vi "Read_Camera_Variant.vi"(8 "error in (no error)":errorcluster, 9 "Variant":variant, 10 "input cluster in":T1 {"Image Type" items=["Grayscale (U8)", "Grayscale (U16)"]; "ROI Parameters"."Size(um)" min=0 max=255 step=0.1 format="%.2f"; "ROI Parameters"."Count" min=0 max=255 step=0.1 format="%.2f"}) -> (0 "error out":errorcluster, 1 "Pixel Size":dbl, 2 "Gain":dbl, 3 "Exposure":dbl, 5 "input cluster out":T1 {"Image Type" items=["Grayscale (U8)", "Grayscale (U16)"]; "ROI Parameters"."Size(um)" min=0 max=255 step=0.1 format="%.2f"; "ROI Parameters"."Count" min=0 max=255 step=0.1 format="%.2f"})   [LabVIEW 2023, in "Camera_Controller.lvlib"]
uses:
  typedefs/ImageProcessingParameters.ctl
  <vilib>/vision/Image Controls.llb/IMAQ Image.ctl
  typedefs/Image Type.ctl
  Camera_Controller.lvlib
  <userlib>/_OpenG.lib/lvdata/lvdata.llb/openg_variant.lvlib
  typedefs/typedefs.lvlib
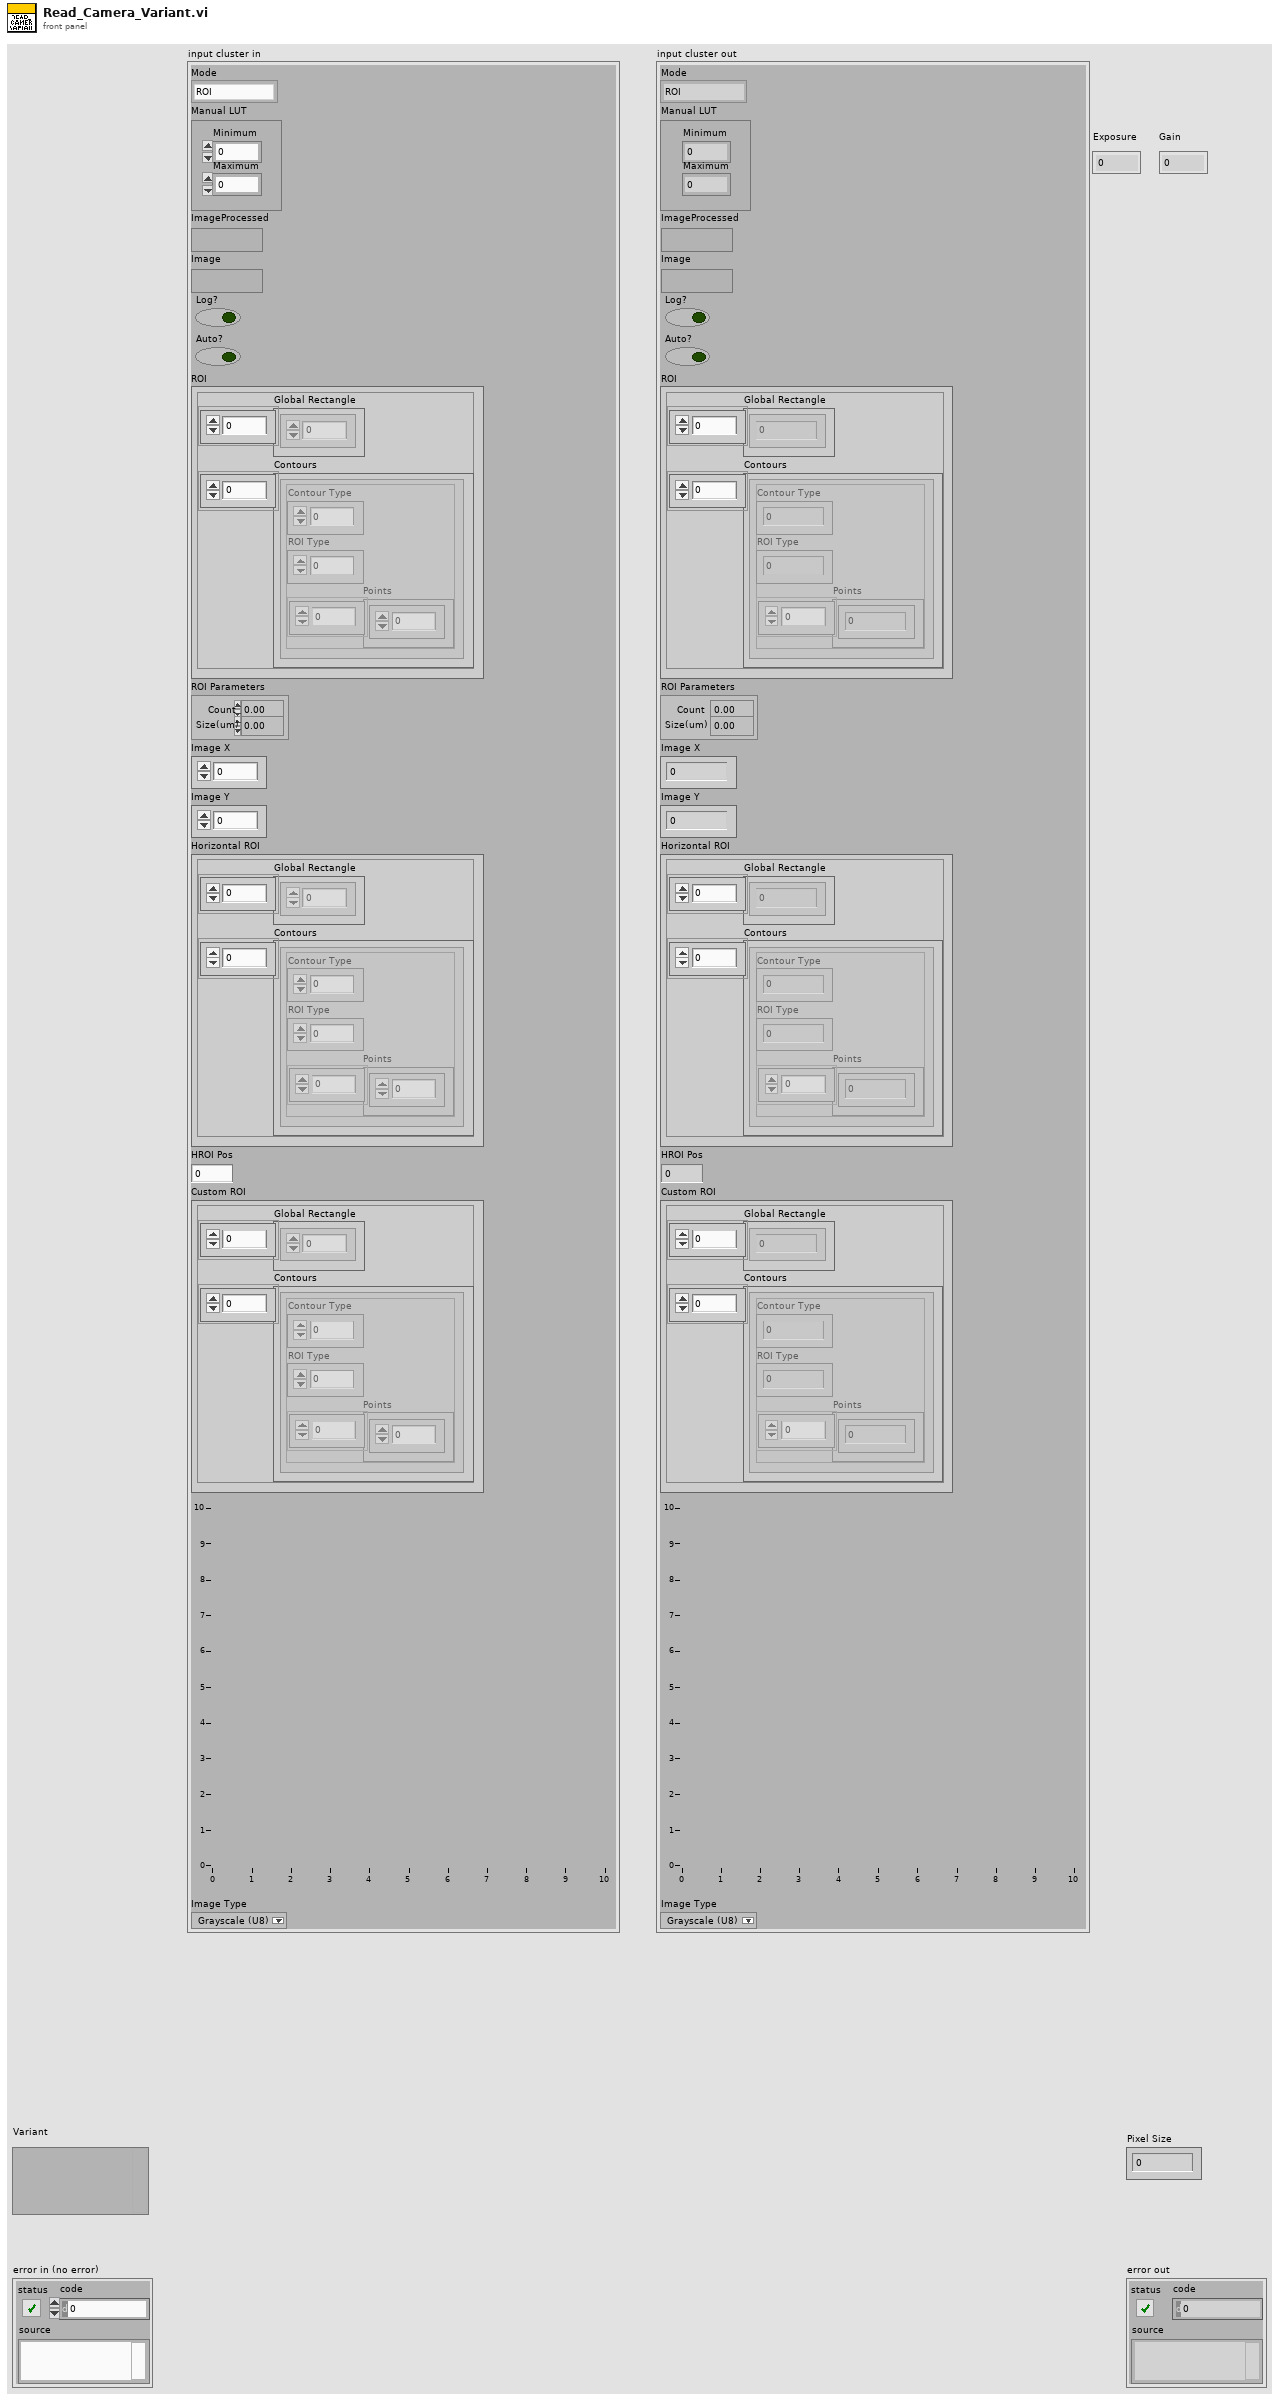
[diagram p1: front panel]
types:
  T1 = typedef "typedefs.lvlib/ImageProcessingParameters.ctl" = cluster{"Mode":enum16{"ROI", "Image"}, "Manual LUT":cluster{"Minimum":dbl, "Maximum":dbl}, "ImageProcessed":T2, "Image ":T2, "Log?":bool, "Auto?":bool, "ROI":cluster{"Global Rectangle":i32[], "Contours":cluster{"Contour Type":u32, "ROI Type":u32, "Points":i32[]}[]}, "ROI Parameters":cluster{"Count":sgl, "Size(um)":sgl}, "Image X":i32, "Image Y":i32, "Horizontal ROI":cluster{"Global Rectangle":i32[], "Contours":cluster{"Contour Type":u32, "ROI Type":u32, "Points":i32[]}[]}, "HROI Pos":u16, "Custom ROI":cluster{"Global Rectangle":i32[], "Contours":cluster{"Contour Type":u32, "ROI Type":u32, "Points":i32[]}[]}, "Intensity Graph":u8[][], "Image Type":T3}
  T2 = typedef "IMAQ Image.ctl" = refnum<image>
  T3 = typedef "typedefs.lvlib/Image Type.ctl" = u32
  T4 = typedef "Image Type" = u32
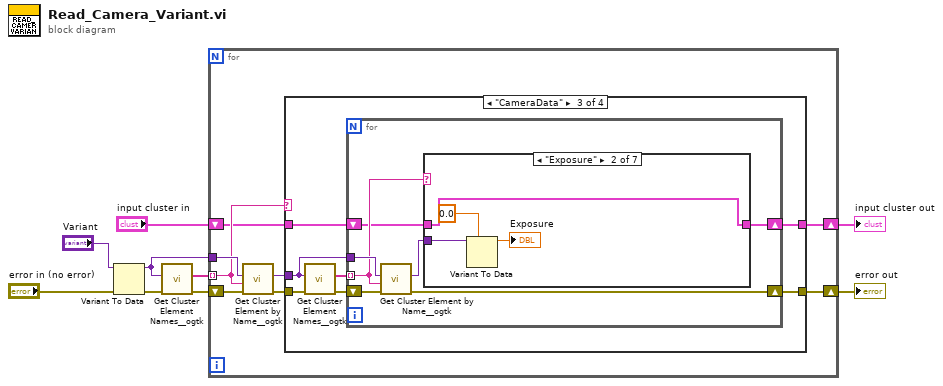
[diagram p0: block diagram]
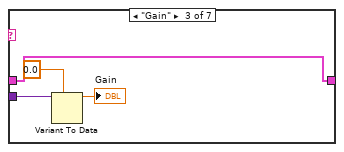
[diagram p5: hidden frame]
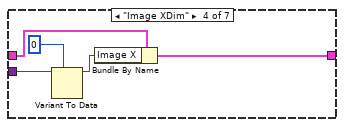
[diagram p6: hidden frame]
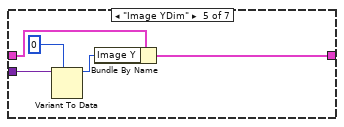
[diagram p7: hidden frame]
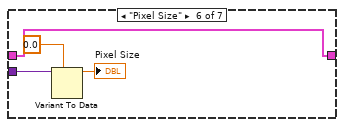
[diagram p8: hidden frame]
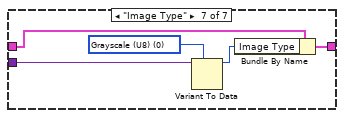
[diagram p9: hidden frame]
diagram:
  n1 = Variant To Data(error in="error in (no error)", Variant="Variant") -> (data=w4:variant, error out=w8:errorcluster)  [unwired: 1 in]
  n2 = call <userlib>:"Get Cluster Element Names__ogtk.vi"("error in (no error)"=w8, "Cluster"=w4) -> ("error out"=w7:errorcluster, "Element Names"=w3:string[])  [unwired: 8 in]
  n3 = for {
    tunnel: w3 -> [w16] mode=indexing
    tunnel: w4 -> [w17]
    shift-right: [w11] -> w9
    shift-left: w7 -> [w12]
    shift-right: [w10] -> w6
    shift-left: "input cluster in" -> [w14]
    n4 = call <userlib>:"Get Cluster Element by Name__ogtk.vi"("error in (no error)"=w12, "Element Name"=w16, "Cluster"=w17) -> ("error out"=w13:errorcluster, "VElement"=w15:variant)  [unwired: 6 in, 1 out]
    n5 = case shown="\"CameraData\"" w16 {
      tunnel: w15 -> [_ _ w27 _]
      tunnel: w14 -> [w19 w21 w26 w65]
      tunnel: [w19 w21 w25 w65] -> w10
      tunnel: w13 -> [w18 w20 w24 w64]
      tunnel: [w18 w20 w22 w64] -> w11
      frame "False", Default {
      }
      frame "InstrError" {
      }
      frame "CameraData" {
        n6 = call <userlib>:"Get Cluster Element Names__ogtk.vi"("error in (no error)"=w24, "Cluster"=w27) -> ("error out"=w23:errorcluster, "Element Names"=w28:string[])  [unwired: 8 in]
        n7 = for {
          tunnel: w28 -> [w34] mode=indexing
          tunnel: w27 -> [w35]
          shift-right: [w29] -> w22
          shift-left: w23 -> [w30]
          shift-right: [w31] -> w25
          shift-left: w26 -> [w32]
          n8 = call <userlib>:"Get Cluster Element by Name__ogtk.vi"("error in (no error)"=w30, "Element Name"=w34, "Cluster"=w35) -> ("error out"=w29:errorcluster, "VElement"=w33:variant)  [unwired: 6 in, 1 out]
          n9 = case shown="\"Exposure\"" w34 {
            tunnel: w33 -> [_ w40 w44 w49 w54 w58 w63]
            tunnel: w32 -> [w36 w37 w42 w47 w51 w55 w62]
            tunnel: [w36 w37 w42 w46 w50 w55 w61] -> w31
            frame "False", Default {
            }
            frame "Exposure" {
              n10 = Variant To Data(type=0.0, Variant=w40) -> (data=→"Exposure":dbl)  [unwired: 1 in, 1 out]
            }
            frame "Gain" {
              n11 = Variant To Data(type=0.0, Variant=w44) -> (data=→"Gain":dbl)  [unwired: 1 in, 1 out]
            }
            frame "Image XDim" {
              n12 = Variant To Data(type=u16 0 ("Image XDim"), Variant=w49) -> (data=w45:u16)  [unwired: 1 in, 1 out]
              n13 = Bundle By Name(cluster=w47, "Image X"=w45) -> (w46:T1)
            }
            frame "Image YDim" {
              n14 = Variant To Data(type=u16 0 ("Image XDim"), Variant=w54) -> (data=w52:u16)  [unwired: 1 in, 1 out]
              n15 = Bundle By Name(cluster=w51, "Image Y"=w52) -> (w50:T1)
            }
            frame "Pixel Size" {
              n16 = Variant To Data(type=0.0 ("Image XDim"), Variant=w58) -> (data=→"Pixel Size":dbl)  [unwired: 1 in, 1 out]
            }
            frame "Image Type" {
              w59 = T4 0 items=["Grayscale (U8)", "Grayscale (I16)", "Grayscale (SGL)", "Complex (CSG)", "RGB (U32)", "HSL (U32)", "RGB (U64)", "Grayscale (U16)"] ("Image Type")
              n17 = Variant To Data(type=w59, Variant=w63) -> (data=w60:T4)  [unwired: 1 in, 1 out]
              n18 = Bundle By Name(cluster=w62, "Image Type"=w60) -> (w61:T1)
            }
          }
        }
      }
      frame "Address" {
      }
    }
  }
  "error out" <- w9
  "input cluster out" <- w6
